vi "Update Mappings by Filter.vi"(8 "error in (no error)":errorcluster, 10 "Destination to Highlight":string, 11 "Loop Data in":T1) -> (0 "error out":errorcluster)   [LabVIEW 2016, in "System Mapping Tool.lvlib"]
uses:
  System Mapping Tool.lvlib
  TypeDefs/Loop Data.ctl
  TypeDefs/UI Refs.ctl
  NationalInstruments.VeriStand.SystemDefinitionAPI
  NationalInstruments.VeriStand.SystemStorageUI
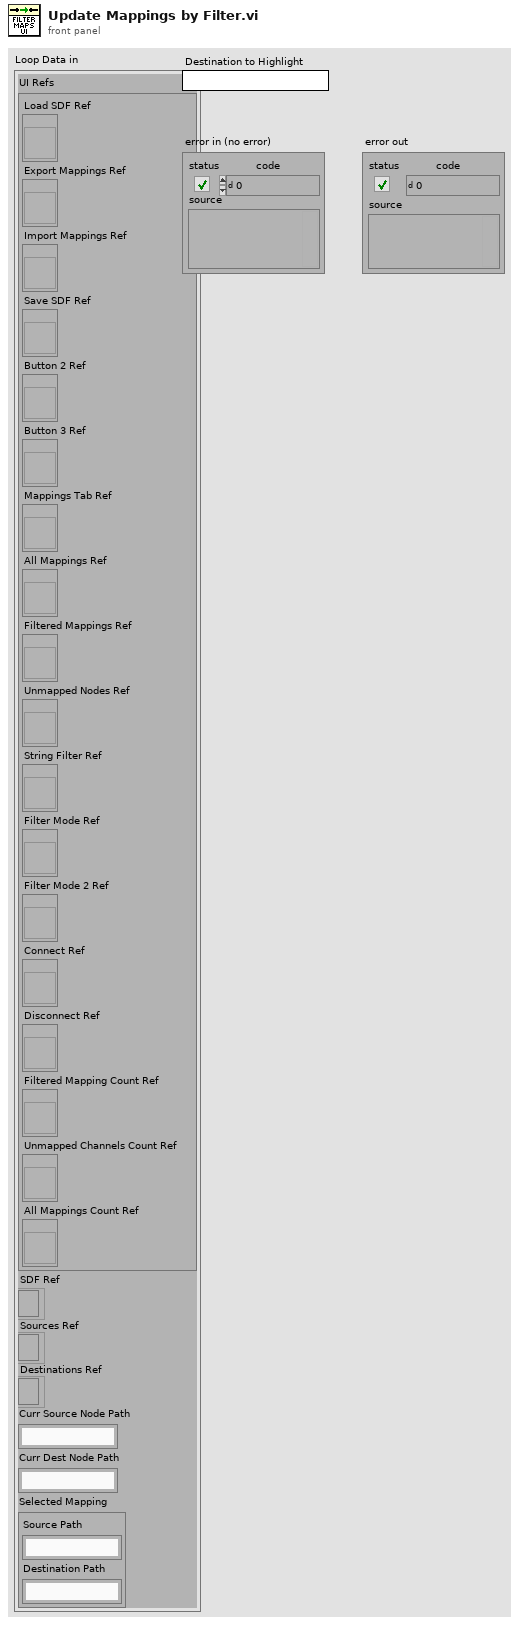
[diagram p1: front panel]
types:
  T1 = typedef "System Mapping Tool.lvlib/Loop Data.ctl" = cluster{"UI Refs":T2, "SDF Ref":refnum<k24>, "Sources Ref":refnum<k24>, "Destinations Ref":refnum<k24>, "Curr Source Node Path":string, "Curr Dest Node Path":string, "Selected Mapping":cluster{"Source Path":string, "Destination Path":string}}
  T2 = typedef "System Mapping Tool.lvlib/UI Refs.ctl" = cluster{"Load SDF Ref":refnum<vi>, "Export Mappings Ref":refnum<vi>, "Import Mappings Ref":refnum<vi>, "Save SDF Ref":refnum<vi>, "Button 2 Ref":refnum<vi>, "Button 3 Ref":refnum<vi>, "Mappings Tab Ref":refnum<vi>, "All Mappings Ref":refnum<vi>, "Filtered Mappings Ref":refnum<vi>, "Unmapped Nodes Ref":refnum<vi>, "String Filter Ref":refnum<vi>, "Filter Mode Ref":refnum<vi>, "Filter Mode 2 Ref":refnum<vi>, "Connect Ref":refnum<vi>, "Disconnect Ref":refnum<vi>, "Filtered Mapping Count Ref":refnum<vi>, "Unmapped Channels Count Ref":refnum<vi>, "All Mappings Count Ref":refnum<vi>}
  T3 = enum32{"All System Mappings", "Filtered Mappings by Node", "Unmapped Channels by Node"}
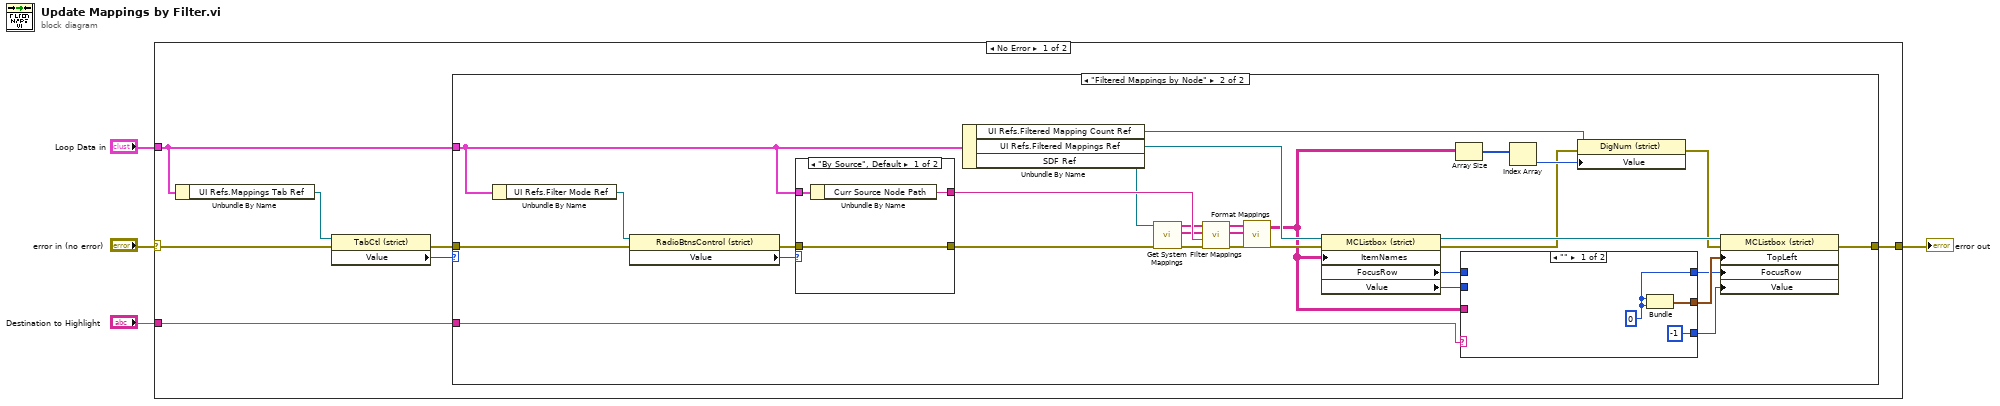
[diagram p0: block diagram]
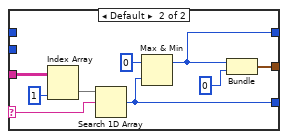
[diagram p3: hidden frame]
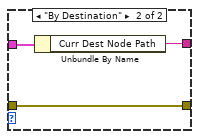
[diagram p4: hidden frame]
diagram:
  n1 = case shown="No Error" "error in (no error)" {
    selector: "error in (no error)" -> [w11 w60]
    tunnel: [w6 w60] -> w3
    tunnel: "Loop Data in" -> [w7 _]
    tunnel: "Destination to Highlight" -> [w5 _]
    frame No Error {
      n2 = Unbundle By Name(w7) -> ("UI Refs.Mappings Tab Ref"=w10:refnum<vi>)
      n3 = property class="TabCtl (strict)"(reference=w10, error in=w11) -> (error out=w8:errorcluster, "Value"=w9:T3)  [unwired: 1 out]
      n4 = case shown="\"Filtered Mappings by Node\"" w9 {
        tunnel: w8 -> [w12 w41]
        tunnel: w7 -> [_ w32]
        tunnel: [w12 w26] -> w6
        tunnel: w5 -> [_ w19]
        frame "All System Mappings", Default {
        }
        frame "Filtered Mappings by Node" {
          n5 = Unbundle By Name(w32) -> ("UI Refs.Filter Mode Ref"=w40:refnum<vi>)
          n6 = property class="RadioBtnsControl (strict)"(reference=w40, error in=w41) -> (error out=w38:errorcluster, "Value"=w39:enum32{"By Source", "By Destination"})  [unwired: 1 out]
          n7 = case shown="\"By Source\", Default" w39 {
            tunnel: w38 -> [w54 w57]
            tunnel: w32 -> [w56 w59]
            tunnel: [w55 w58] -> w36
            tunnel: [w54 w57] -> w37
            frame "By Source", Default {
              n8 = Unbundle By Name(w56) -> ("Curr Source Node Path"=w55:string)
            }
            frame "By Destination" {
              n9 = Unbundle By Name(w59) -> ("Curr Dest Node Path"=w58:string)
            }
          }
          n10 = Unbundle By Name(w32) -> ("UI Refs.Filtered Mapping Count Ref"=w16:refnum<vi>, "UI Refs.Filtered Mappings Ref"=w31:refnum<vi>, "SDF Ref"=w27:refnum<k24>)
          n11 = call "Get System Mappings.vi"("error in (no error)"=w37, "SDF Ref"=w27) -> ("error out"=w33:errorcluster, "Destinations"=w34:string[], "Sources"=w35:string[])  [unwired: 7 in]
          n12 = call "Filter Mappings.vi"("error in (no error)"=w33, "Path to Filter"=w36, "Destinations"=w34, "Sources"=w35) -> ("error out"=w30:errorcluster, "Filtered Destinations"=w28:string[], "Filtered Sources"=w29:string[])  [unwired: 5 in]
          n13 = call "Format Mappings.vi"("Destinations"=w28, "Sources"=w29) -> ("Mappings"=w15:string[][])  [unwired: 3 in]
          n14 = property class="MCListbox (strict)"(reference=w31, error in=w30, "ItemNames"=w15) -> (reference out=w25:refnum<vi>, error out=w14:errorcluster, "FocusRow"=w24:i32, "Value"=w20:i32)
          n15 = Array Size(array=w15) -> (size(s)=w18:i32[])
          n16 = case shown="\"\"" w19 {
            selector: w19 -> [_ w49]
            tunnel: [w44 w48] -> w23
            tunnel: w15 -> [_ w52]
            tunnel: w24 -> [_ _]
            tunnel: [w42 w47] -> w21
            tunnel: [-1 ("index of element") w45] -> w22
            tunnel: w20 -> [_ _]
            frame "" {
              w42 = 0
              n17 = Bundle(w42, w42) -> (w44:cluster{i32, i32})  [unwired: 1 in]
            }
            frame Default {
              n18 = Index Array(array=w52, index (col)=1 ("disabled index (col)")) -> (element=w51:string[])  [unwired: 1 in]
              n19 = Search 1D Array(1D array=w51, element=w49) -> (index of element=w45:i32)  [unwired: 1 in]
              n20 = Max & Min(x=0, y=w45) -> (max(x,y)=w47:i32)  [unwired: 1 out]
              n21 = Bundle(w47, 0) -> (w48:cluster{i32, i32})  [unwired: 1 in]
            }
          }
          n22 = Index Array(array=w18) -> (element=w17:i32)  [unwired: 1 in]
          n23 = property class="DigNum (strict)"(reference=w16, error in=w14, "Value"=w17) -> (error out=w13:errorcluster)  [unwired: 1 out]
          n24 = property class="MCListbox (strict)"(reference=w25, error in=w13, "TopLeft"=w23, "FocusRow"=w21, "Value"=w22) -> (error out=w26:errorcluster)  [unwired: 1 out]
        }
      }
    }
    frame Error {
    }
  }
  "error out" <- w3
